vi "control motor.vi"(12 "error in":errorcluster) -> (14 "error out":errorcluster)   [LabVIEW 2018]
uses:
  <vilib>/DAQmx/read.llb/DAQmx Read (Analog 1D Wfm NChan NSamp).vi
  <vilib>/DAQmx/write.llb/DAQmx Write (Digital 1D Bool NChan 1Samp 1Line).vi
  <vilib>/DAQmx/write.llb/DAQmx Write (Analog 1D DBL NChan 1Samp).vi
  <vilib>/DAQmx/create/channels.llb/DAQmx Create Channel (AI-Voltage-Basic).vi
  <vilib>/DAQmx/configure/timing.llb/DAQmx Timing (Sample Clock).vi
  <vilib>/DAQmx/miscellaneous.llb/DAQmx Fill In Error Info.vi
  <vilib>/DAQmx/create/channels.llb/DAQmx Create Channel (DO-Digital Output).vi
  <vilib>/DAQmx/create/channels.llb/DAQmx Create Channel (AO-Voltage-Basic).vi
  <resource>/objmgr/daqmx.rc
panel:
  out "data for motor":bool[](array[boolean])=[TRUE, FALSE, TRUE, FALSE, TRUE, FALSE, TRUE, FALSE]
  out "cycles ran":i16=40
  out "cycles ran":i16
  out "cycles ran":i16
  out "cycles ran":i16
  in  "Station 4":bool=TRUE
  in  "Station 3":bool=TRUE
  in  "Station 2":bool=TRUE
  in  "Station1":bool=TRUE
  in  "Cycles":i16=2500
  in  "Cycles":i16=2500
  in  "Cycles":i16=2500
  in  "Cycles":i16=2500
  in  "stop":bool
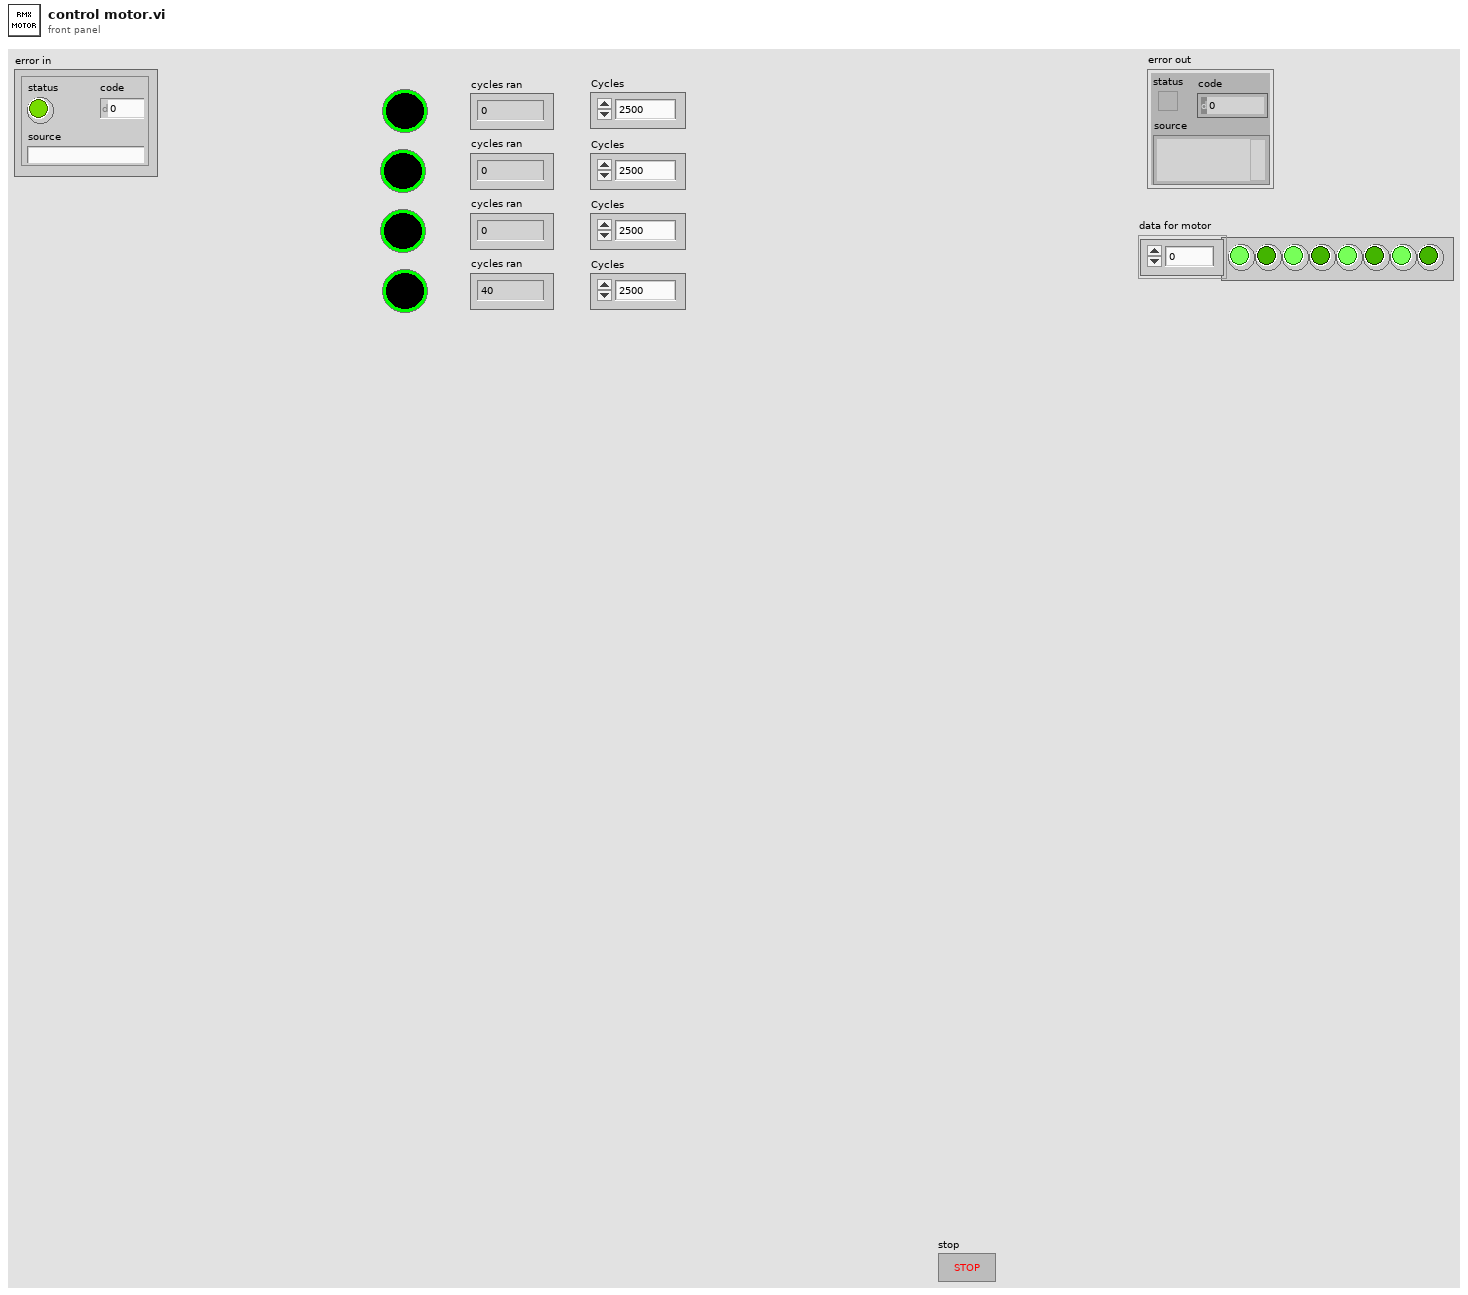
[diagram p1: front panel]
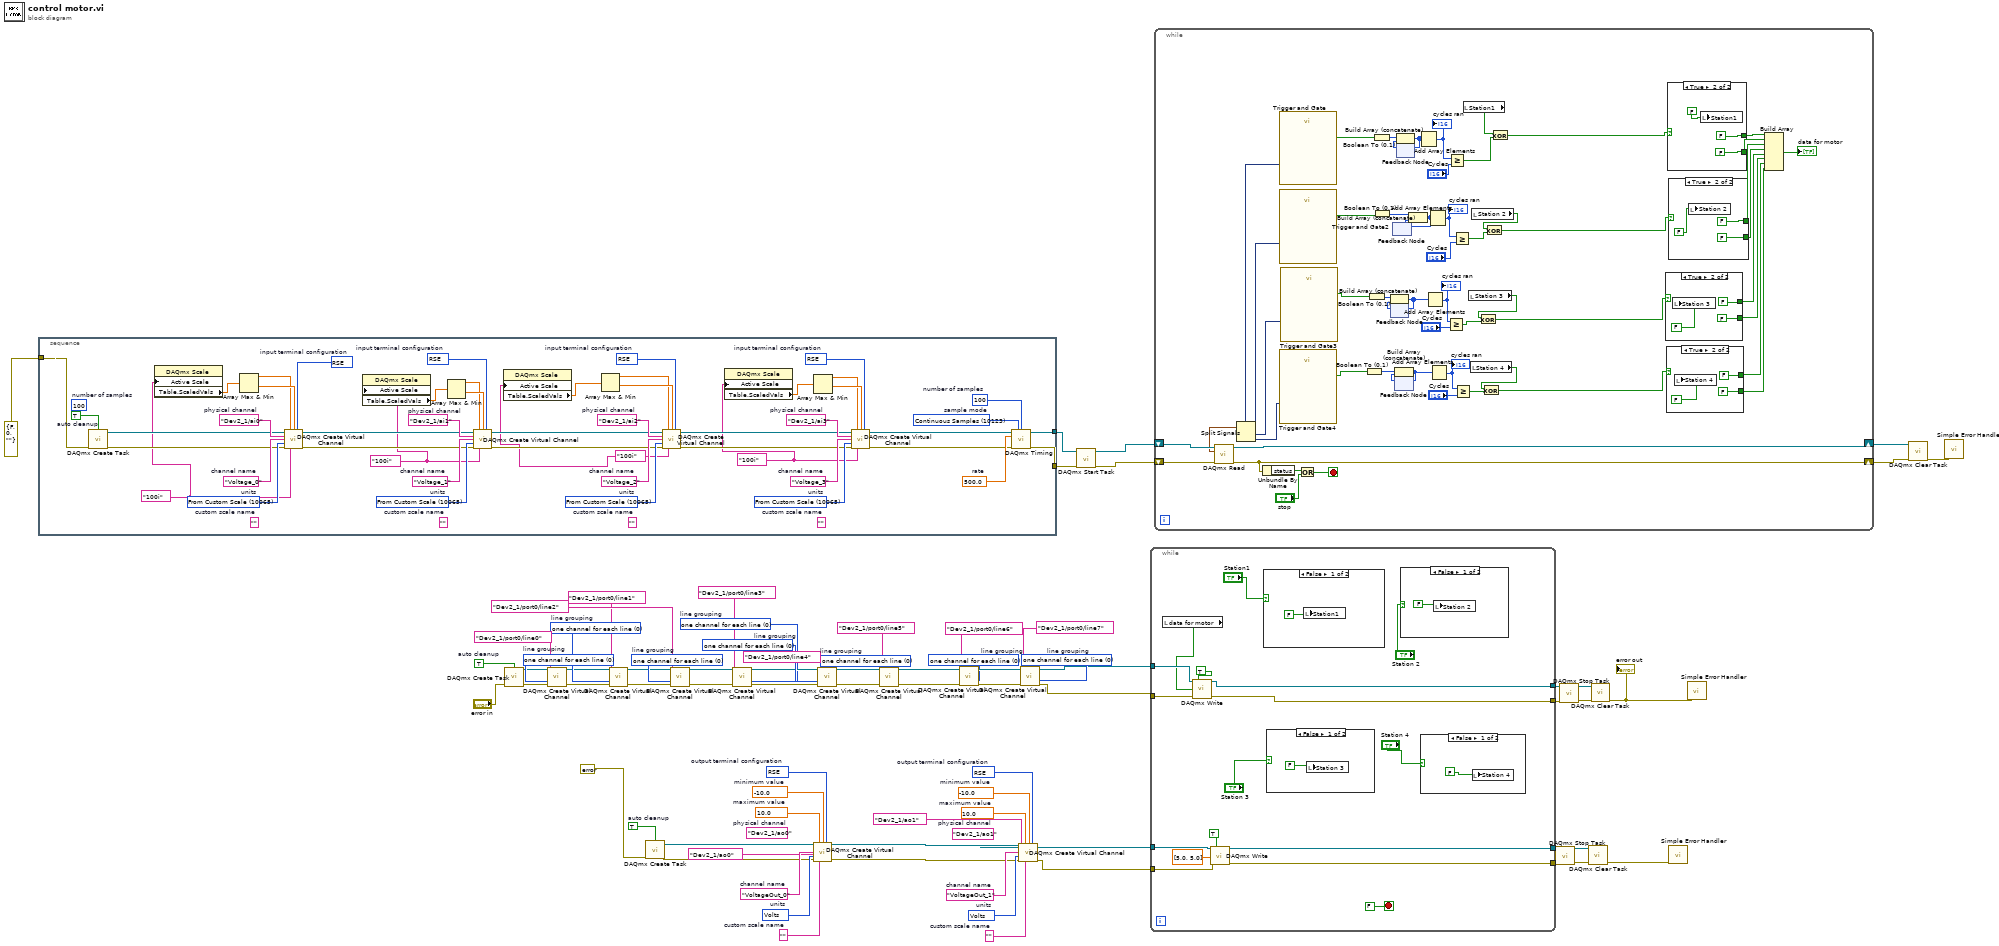
[diagram p0: block diagram]
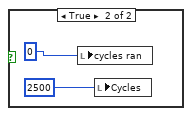
[diagram p2: hidden frame]
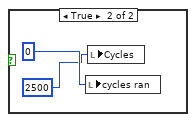
[diagram p3: hidden frame]
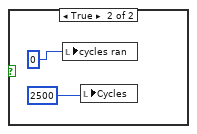
[diagram p4: hidden frame]
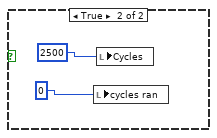
[diagram p5: hidden frame]
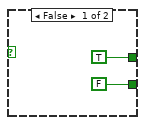
[diagram p6: hidden frame]
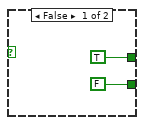
[diagram p7: hidden frame]
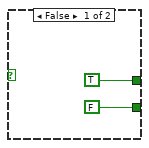
[diagram p8: hidden frame]
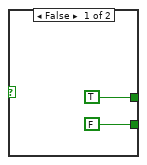
[diagram p9: hidden frame]
diagram:
  (unwired) 100  # number of samples
  w35 = 10083 items=["Default"=-1, "RSE"=10083, "Differential"=10106, "Pseudodifferential"=12529]  # output terminal configuration
  w34 = 10348 items=["Volts"=10348, "From Custom Scale"=10065]  # units
  w33 = "VoltageOut_1"  # channel name
  w32 = ""  # custom scale name
  w31 = -10.0  # minimum value
  w30 = 10.0  # maximum value
  (unwired) "Dev2_1/ao1"  # physical channel
  w28 = 10083 items=["Default"=-1, "RSE"=10083, "Differential"=10106, "Pseudodifferential"=12529]  # output terminal configuration
  w27 = 10348 items=["Volts"=10348, "From Custom Scale"=10065]  # units
  w26 = "VoltageOut_0"  # channel name
  w24 = ""  # custom scale name
  w23 = -10.0  # minimum value
  w22 = 10.0  # maximum value
  (unwired) "Dev2_1/ao0"  # physical channel
  w20 = TRUE  # auto cleanup
  w75 = 0 items=["one channel for each line", "one channel for all lines"]  # line grouping
  w72 = 0 items=["one channel for each line", "one channel for all lines"]  # line grouping
  w69 = 0 items=["one channel for each line", "one channel for all lines"]  # line grouping
  w66 = 0 items=["one channel for each line", "one channel for all lines"]  # line grouping
  w63 = 0 items=["one channel for each line", "one channel for all lines"]  # line grouping
  w60 = 0 items=["one channel for each line", "one channel for all lines"]  # line grouping
  w57 = 0 items=["one channel for each line", "one channel for all lines"]  # line grouping
  w54 = 0 items=["one channel for each line", "one channel for all lines"]  # line grouping
  w52 = TRUE  # auto cleanup
  n1 = stacked-sequence {
    tunnel: errorcluster {"status"=FALSE, "code"=0, "source"=""} ("error in") -> [w95]
    tunnel: [w78] -> w10
    tunnel: [w77] -> w9
    frame #0 {
      w82 = tag "100i" ("custom scale name 3")
      w86 = tag "100i" ("custom scale name 2")
      w90 = tag "100i" ("custom scale name")
      w94 = tag "100i" ("custom scale name")
      w125 = 10123 items=["Finite Samples"=10178, "Continuous Samples"=10123, "Hardware Timed Single Point"=12522]  # sample mode
      w124 = 100  # number of samples
      w123 = 500.0  # rate
      w121 = 10083 items=["default"=-1, "RSE"=10083, "NRSE"=10078, "Differential"=10106, "Pseudodifferential"=12529]  # input terminal configuration
      w120 = 10065 items=["Volts"=10348, "From Custom Scale"=10065]  # units
      w119 = "Voltage_3"  # channel name
      (unwired) ""  # custom scale name
      w117 = "Dev2_1/ai3"  # physical channel
      w115 = 10083 items=["default"=-1, "RSE"=10083, "NRSE"=10078, "Differential"=10106, "Pseudodifferential"=12529]  # input terminal configuration
      w114 = 10065 items=["Volts"=10348, "From Custom Scale"=10065]  # units
      w113 = "Voltage_2"  # channel name
      (unwired) ""  # custom scale name
      w111 = "Dev2_1/ai2"  # physical channel
      w109 = 10083 items=["default"=-1, "RSE"=10083, "NRSE"=10078, "Differential"=10106, "Pseudodifferential"=12529]  # input terminal configuration
      w108 = 10065 items=["Volts"=10348, "From Custom Scale"=10065]  # units
      w107 = "Voltage_1"  # channel name
      (unwired) ""  # custom scale name
      w105 = "Dev2_1/ai1"  # physical channel
      w103 = 10083 items=["default"=-1, "RSE"=10083, "NRSE"=10078, "Differential"=10106, "Pseudodifferential"=12529]  # input terminal configuration
      w102 = 10065 items=["Volts"=10348, "From Custom Scale"=10065]  # units
      w101 = "Voltage_0"  # channel name
      (unwired) ""  # custom scale name
      w99 = "Dev2_1/ai0"  # physical channel
      w97 = TRUE  # auto cleanup
      n2 = call <vilib>:"DAQmx Create Task.vi"("auto cleanup"=w97, "error in"=w95) -> ("task out"=w98:refnum<k21>, "error out"=w96:errorcluster)  [unwired: 12 in]
      n3 = property class="DAQmx Scale"("Active Scale"=w94) -> ("Table.ScaledVals"=w93:dbl[])  [unwired: 2 in, 2 out]
      n4 = Array Max & Min(array=w93) -> (max value=w91:dbl, min value=w92:dbl)  [unwired: 2 out]
      n5 = call-poly <vilib>:"DAQmx Create Virtual Channel.vi"("task in"=w98, "maximum value"=w91, "minimum value"=w92, "input terminal configuration"=w103, "physical channels"=w99, "name to assign"=w101, "units"=w102, "error in"=w96, "custom scale name"=w94) -> ("task out"=w104:refnum<k21>, "error out"=w100:errorcluster)  [unwired: 5 in]
      n6 = property class="DAQmx Scale"("Active Scale"=w90) -> ("Table.ScaledVals"=w89:dbl[])  [unwired: 2 in, 2 out]
      n7 = Array Max & Min(array=w89) -> (max value=w87:dbl, min value=w88:dbl)  [unwired: 2 out]
      n8 = call-poly <vilib>:"DAQmx Create Virtual Channel.vi"("task in"=w104, "maximum value"=w87, "minimum value"=w88, "input terminal configuration"=w109, "physical channels"=w105, "name to assign"=w107, "units"=w108, "error in"=w100, "custom scale name"=w90) -> ("task out"=w110:refnum<k21>, "error out"=w106:errorcluster)  [unwired: 5 in]
      n9 = property class="DAQmx Scale"("Active Scale"=w86) -> ("Table.ScaledVals"=w85:dbl[])  [unwired: 2 in, 2 out]
      n10 = Array Max & Min(array=w85) -> (max value=w83:dbl, min value=w84:dbl)  [unwired: 2 out]
      n11 = call-poly <vilib>:"DAQmx Create Virtual Channel.vi"("task in"=w110, "maximum value"=w83, "minimum value"=w84, "input terminal configuration"=w115, "physical channels"=w111, "name to assign"=w113, "units"=w114, "error in"=w106, "custom scale name"=w86) -> ("task out"=w116:refnum<k21>, "error out"=w112:errorcluster)  [unwired: 5 in]
      n12 = property class="DAQmx Scale"("Active Scale"=w82) -> ("Table.ScaledVals"=w81:dbl[])  [unwired: 2 in, 2 out]
      n13 = Array Max & Min(array=w81) -> (max value=w79:dbl, min value=w80:dbl)  [unwired: 2 out]
      n14 = call-poly <vilib>:"DAQmx Create Virtual Channel.vi"("task in"=w116, "maximum value"=w79, "minimum value"=w80, "input terminal configuration"=w121, "physical channels"=w117, "name to assign"=w119, "units"=w120, "error in"=w112, "custom scale name"=w82) -> ("task out"=w122:refnum<k21>, "error out"=w118:errorcluster)  [unwired: 5 in]
      n15 = call-poly <vilib>:"DAQmx Timing.vi"("task/channels in"=w122, "sample mode"=w125, "samples per channel"=w124, "rate"=w123, "error in"=w118) -> ("task out"=w78:refnum<k21>, "error out"=w77:errorcluster)  [unwired: 9 in]
    }
  }
  n16 = call <vilib>:"DAQmx Create Task.vi"("auto cleanup"=w52, "error in"="error in") -> ("task out"=w53:refnum<k21>, "error out"=w51:errorcluster)  [unwired: 12 in]
  n17 = call-poly <vilib>:"DAQmx Create Virtual Channel.vi"("task in"=w53, "lines"=tag "Dev2_1/port0/line0" ("lines 1"), "line grouping"=w54, "error in"=w51) -> ("task out"=w56:refnum<k21>, "error out"=w55:errorcluster)  [unwired: 10 in]
  n18 = call-poly <vilib>:"DAQmx Create Virtual Channel.vi"("task in"=w56, "lines"=tag "Dev2_1/port0/line1" ("lines 2"), "line grouping"=w57, "error in"=w55) -> ("task out"=w59:refnum<k21>, "error out"=w58:errorcluster)  [unwired: 10 in]
  n19 = call <vilib>:"DAQmx Create Task.vi"("auto cleanup"=w20, "error in"=errorcluster {"status"=FALSE, "code"=0, "source"=""}) -> ("task out"=w21:refnum<k21>, "error out"=w19:errorcluster)  [unwired: 12 in]
  n20 = call-poly <vilib>:"DAQmx Create Virtual Channel.vi"("task in"=w59, "lines"=tag "Dev2_1/port0/line2" ("lines 3"), "line grouping"=w60, "error in"=w58) -> ("task out"=w62:refnum<k21>, "error out"=w61:errorcluster)  [unwired: 10 in]
  n21 = call-poly <vilib>:"DAQmx Create Virtual Channel.vi"("task in"=w62, "lines"=tag "Dev2_1/port0/line3" ("lines4"), "line grouping"=w63, "error in"=w61) -> ("task out"=w65:refnum<k21>, "error out"=w64:errorcluster)  [unwired: 10 in]
  n22 = call-poly <vilib>:"DAQmx Create Virtual Channel.vi"("task in"=w21, "maximum value"=w22, "minimum value"=w23, "output terminal configuration"=w28, "physical channels"=tag "Dev2_1/ao0", "name to assign"=w26, "units"=w27, "error in"=w19, "custom scale name"=w24) -> ("task out"=w29:refnum<k21>, "error out"=w25:errorcluster)  [unwired: 5 in]
  n23 = call-poly <vilib>:"DAQmx Create Virtual Channel.vi"("task in"=w65, "lines"=tag "Dev2_1/port0/line4" ("lines 5"), "line grouping"=w66, "error in"=w64) -> ("task out"=w68:refnum<k21>, "error out"=w67:errorcluster)  [unwired: 10 in]
  n24 = call-poly <vilib>:"DAQmx Create Virtual Channel.vi"("task in"=w68, "lines"=tag "Dev2_1/port0/line5" ("lines 6"), "line grouping"=w69, "error in"=w67) -> ("task out"=w71:refnum<k21>, "error out"=w70:errorcluster)  [unwired: 10 in]
  n25 = call-poly <vilib>:"DAQmx Create Virtual Channel.vi"("task in"=w71, "lines"=tag "Dev2_1/port0/line6" ("lines 7"), "line grouping"=w72, "error in"=w70) -> ("task out"=w74:refnum<k21>, "error out"=w73:errorcluster)  [unwired: 10 in]
  n26 = call-poly <vilib>:"DAQmx Create Virtual Channel.vi"("task in"=w29, "maximum value"=w30, "minimum value"=w31, "output terminal configuration"=w35, "physical channels"=tag "Dev2_1/ao1" ("physical channels 2"), "name to assign"=w33, "units"=w34, "error in"=w25, "custom scale name"=w32) -> ("task out"=w8:refnum<k21>, "error out"=w7:errorcluster)  [unwired: 5 in]
  n27 = call-poly <vilib>:"DAQmx Create Virtual Channel.vi"("task in"=w74, "lines"=tag "Dev2_1/port0/line7" ("lines 8"), "line grouping"=w75, "error in"=w73) -> ("task out"=w6:refnum<k21>, "error out"=w5:errorcluster)  [unwired: 10 in]
  n28 = call <vilib>:"DAQmx Start Task.vi"("task/channels in"=w10, "error in"=w9) -> ("task out"=w16:refnum<k21>, "error out"=w15:errorcluster)  [unwired: 12 in]
  n29 = while {
    tunnel: w8 -> [w142]
    tunnel: w7 -> [w139]
    tunnel: w6 -> [w138]
    tunnel: w5 -> [w136]
    tunnel: [w134] -> w4
    tunnel: [w133] -> w3
    tunnel: [w132] -> w2
    tunnel: [w131] -> w1
    stop <- FALSE stop-if-true
    n30 = local read "data for motor"() -> (w135:bool[])
    n31 = call-poly <vilib>:"DAQmx Write.vi"("task/channels in"=w138, "auto start"=TRUE, "data"=w135, "error in"=w136) -> ("task out"=w132:refnum<k21>, "error out"=w131:errorcluster)  [unwired: 9 in, 1 out]
    n32 = call-poly <vilib>:"DAQmx Write.vi"("task/channels in"=w142, "auto start"=TRUE, "data"=dbl[] [5.0, 5.0] ("Speed"), "error in"=w139) -> ("task out"=w134:refnum<k21>, "error out"=w133:errorcluster)  [unwired: 9 in, 1 out]
    n33 = case shown="False" "Station1" {
      frame False {
        n34 = local write "Station1"(FALSE) -> ()
      }
      frame True {
        n35 = local write "cycles ran"(0) -> ()
        n36 = local write "Cycles"(2500) -> ()
      }
    }
    n37 = case shown="False" "Station 3" {
      frame False {
        n38 = local write "Station 3"(FALSE) -> ()
      }
      frame True {
        n39 = local write "cycles ran"(0) -> ()
        n40 = local write "Cycles"(2500) -> ()
      }
    }
    n41 = case shown="False" "Station 2" {
      frame False {
        n42 = local write "Station 2"(FALSE) -> ()
      }
      frame True {
        n43 = local write "cycles ran"(0) -> ()
        n44 = local write "Cycles"(2500) -> ()
      }
    }
    n45 = case shown="False" "Station 4" {
      frame False {
        n46 = local write "Station 4"(FALSE) -> ()
      }
      frame True {
        n47 = local write "cycles ran"(0) -> ()
        n48 = local write "Cycles"(2500) -> ()
      }
    }
  }
  n49 = while {
    shift-right: [w208] -> w13
    shift-left: w16 -> [w211]
    shift-right: [w209] -> w14
    shift-left: w15 -> [w210]
    stop <- w200 stop-if-true
    n50 = call-poly <vilib>:"DAQmx Read.vi"("task/channels in"=w211, "error in"=w210) -> ("task out"=w208:refnum<k21>, "data"=w205:waveform(dbl)[], "error out"=w209:errorcluster)  [unwired: 11 in]
    n51 = Split Signals(w205) -> (w204:dynamicdata, w203:dynamicdata, w202:dynamicdata, w201:dynamicdata)  [unwired: 4 in]
    n52 = Unbundle By Name(w209) -> ("status"=w207:bool)
    n53 = call "Trigger and Gate"("Signals"=w204) -> ("Data Available"=w199:bool)  [unwired: 7 in, 3 out]
    n54 = call "Trigger and Gate2"("Signals"=w203) -> ("Data Available"=w188:bool)  [unwired: 7 in, 3 out]
    n55 = call "Trigger and Gate4"("Signals"=w201) -> ("Data Available"=w176:bool)  [unwired: 7 in, 3 out]
    n56 = call "Trigger and Gate3"("Signals"=w202) -> ("Data Available"=w183:bool)  [unwired: 7 in, 3 out]
    n57 = Or(x=w207, y="stop") -> (x .or. y?=w200:bool)
    n58 = Boolean To (0,1)(Boolean=w176) -> (0, 1=w179:i16)
    n59 = Boolean To (0,1)(Boolean=w183) -> (0, 1=w184:i16)
    n60 = Boolean To (0,1)(Boolean=w199) -> (0, 1=w198:i16)
    n61 = Boolean To (0,1)(Boolean=w188) -> (0, 1=w191:i16)
    n62 = feedback #1() -> (w185:i16[])  [unwired: 1 in]
    n63 = Build Array (concatenate)(w184, w185) -> (w186:i16[])
    n64 = feedback-in #1(w186) -> ()
    n65 = feedback #2() -> (w190:i16[])  [unwired: 1 in]
    n66 = feedback #3() -> (w178:i16[])  [unwired: 1 in]
    n67 = Build Array (concatenate)(w179, w178) -> (w177:i16[])
    n68 = feedback-in #3(w177) -> ()
    n69 = feedback #4() -> (w197:i16[])  [unwired: 1 in]
    n70 = Build Array (concatenate)(w198, w197) -> (w196:i16[])
    n71 = feedback-in #4(w196) -> ()
    n72 = Build Array (concatenate)(w191, w190) -> (w189:i16[])
    n73 = feedback-in #2(w189) -> ()
    n74 = Add Array Elements(numeric array=w196) -> (sum=w194:i16)
    "cycles ran" <- w194
    n75 = Add Array Elements(numeric array=w186) -> (sum=w182:i16)
    "cycles ran" <- w182
    n76 = Add Array Elements(numeric array=w189) -> (sum=w193:i16)
    "cycles ran" <- w193
    n77 = Add Array Elements(numeric array=w177) -> (sum=w181:i16)
    "cycles ran" <- w181
    n78 = Greater Or Equal?(x=w182, y="Cycles") -> (x >= y?=w172:bool)
    n79 = Greater Or Equal?(x=w194, y="Cycles") -> (x >= y?=w160:bool)
    n80 = Greater Or Equal?(x=w193, y="Cycles") -> (x >= y?=w175:bool)
    n81 = Greater Or Equal?(x=w181, y="Cycles") -> (x >= y?=w170:bool)
    n82 = local read "Station1"() -> (w159:bool)
    n83 = local read "Station 3"() -> (w173:bool)
    n84 = local read "Station 4"() -> (w171:bool)
    n85 = local read "Station 2"() -> (w174:bool)
    n86 = Exclusive Or(1:w172, 2:w173) -> (0:w157:bool)
    n87 = Exclusive Or(1:w170, 2:w171) -> (0:w158:bool)
    n88 = Exclusive Or(1:w175, 2:w174) -> (0:w156:bool)
    n89 = Exclusive Or(1:w160, 2:w159) -> (0:w155:bool)
    n90 = case shown="True" w157 {
      tunnel: [TRUE FALSE] -> w165
      tunnel: [FALSE FALSE] -> w164
      frame False {
      }
      frame True {
        n91 = local write "Station 3"(FALSE) -> ()
      }
    }
    n92 = case shown="True" w158 {
      tunnel: [TRUE FALSE] -> w163
      tunnel: [FALSE FALSE] -> w162
      frame False {
      }
      frame True {
        n93 = local write "Station 4"(FALSE) -> ()
      }
    }
    n94 = case shown="True" w155 {
      tunnel: [TRUE FALSE] -> w169
      tunnel: [FALSE FALSE] -> w168
      frame False {
      }
      frame True {
        n95 = local write "Station1"(FALSE) -> ()
      }
    }
    n96 = case shown="True" w156 {
      tunnel: [TRUE FALSE] -> w167
      tunnel: [FALSE FALSE] -> w166
      frame False {
      }
      frame True {
        n97 = local write "Station 2"(FALSE) -> ()
      }
    }
    n98 = Build Array(w169, w168, w167, w166, w165, w164, w163, w162) -> (→"data for motor":bool[])
  }
  n99 = call <vilib>:"DAQmx Stop Task.vi"("task/channels in"=w4, "error in"=w3) -> ("task out"=w40:refnum<k21>, "error out"=w39:errorcluster)  [unwired: 12 in]
  n100 = call <vilib>:"DAQmx Stop Task.vi"("task/channels in"=w2, "error in"=w1) -> ("task out"=w42:refnum<k21>, "error out"=w41:errorcluster)  [unwired: 12 in]
  n101 = call <vilib>:"DAQmx Clear Task.vi"("task in"=w40, "error in"=w39) -> ("error out"=w37:errorcluster)  [unwired: 13 in]
  n102 = call <vilib>:"DAQmx Clear Task.vi"("task in"=w42, "error in"=w41) -> ("error out"=w38:errorcluster)  [unwired: 13 in]
  "error out" <- w38
  n103 = call <vilib>:"Simple Error Handler.vi"("error in (no error)"=w37) -> ()  [unwired: 4 in, 5 out]
  n104 = call <vilib>:"Simple Error Handler.vi"("error in (no error)"=w38) -> ()  [unwired: 4 in, 5 out]
  n105 = call <vilib>:"DAQmx Clear Task.vi"("task in"=w13, "error in"=w14) -> ("error out"=w11:errorcluster)  [unwired: 13 in]
  n106 = call <vilib>:"Simple Error Handler.vi"("error in (no error)"=w11) -> ()  [unwired: 4 in, 5 out]
